vi "SMU2400Init.vi"(7 "Keithley Config":T1={"Source Compliance"=0.1, "Min Voltage"=0.0, "Max Voltage"=5.0, "Source Mode"=0, "Number of Points"=50} {"Source Mode" items=["Voltage", "Current"]}, 8 "error in (no error)":errorcluster, 11 "Keithley 2400 Name":refnum<visa-resource-name>) -> (0 "error out":errorcluster, 3 "VISA resource name out":refnum<visa-resource-name>)   [LabVIEW 2020, in "SMU.lvclass"]
uses:
  SMU.lvclass
  typeDefs/keithleySettings.ctl
  <instrlib>/Keithley 24XX/Keithley 24XX.lvlib
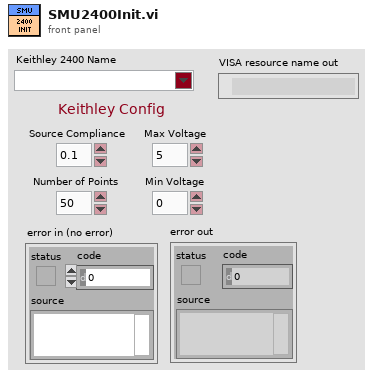
[diagram p1: front panel]
types:
  T1 = typedef "keithleySettings.ctl" = cluster{"Source Compliance":dbl, "Min Voltage":dbl, "Max Voltage":dbl, "Source Mode":u16, "Number of Points":u32}
  T2 = cluster{"Baud Rate":u32, "Parity":u16, "Data Bits":u16, "Stop Bits":u16, "Flow Control":u16}
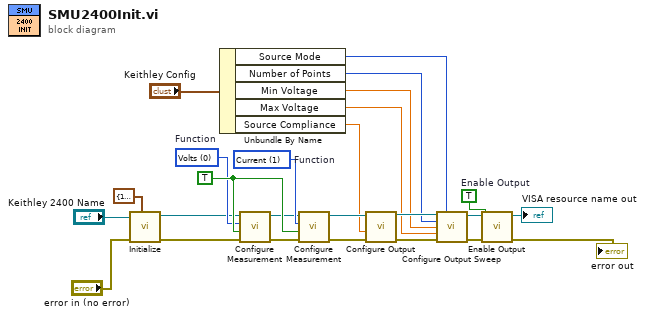
[diagram p0: block diagram]
diagram:
  w22 = TRUE  # Enable Output
  w17 = TRUE ("Enable Auto Range")
  w16 = u16 1 items=["Volts", "Current", "Resistance"]  # Function
  w15 = u16 0 items=["Volts", "Current", "Resistance"]  # Function
  n1 = call <instrlib>:"Initialize.vi"("Serial Configuration"=T2 {"Baud Rate"=19200, "Parity"=0, "Data Bits"=8, "Stop Bits"=10, "Flow Control"=0}, "error in (no error)"="error in (no error)", "VISA resource name"="Keithley 2400 Name") -> ("error out"=w12:errorcluster, "VISA resource name out"=w11:refnum<visa-resource-name>)  [unwired: 7 in]
  n2 = Unbundle By Name("Keithley Config") -> ("Source Mode"=w5:u16, "Number of Points"=w7:u32, "Min Voltage"=w8:dbl, "Max Voltage"=w9:dbl, "Source Compliance"=w4:dbl)
  n3 = call <instrlib>:"Configure Measurement.vi"("error in (no error)"=w12, "Enable Auto Range (T:Enable)"=w17, "Function (0: Volts)"=w15, "VISA resource name"=w11) -> ("error out"=w13:errorcluster, "VISA resource name out"=w14:refnum<visa-resource-name>)  [unwired: 6 in]
  n4 = call <instrlib>:"Configure Measurement.vi"("error in (no error)"=w13, "Enable Auto Range (T:Enable)"=w17, "Function (0: Volts)"=w16, "VISA resource name"=w14) -> ("error out"=w24:errorcluster, "VISA resource name out"=w23:refnum<visa-resource-name>)  [unwired: 6 in]
  n5 = call <instrlib>:"Configure Output.vi"("error in (no error)"=w24, "Compliance  Level (0.1)"=w4, "VISA resource name"=w23) -> ("error out"=w18:errorcluster, "VISA resource name out"=w19:refnum<visa-resource-name>)  [unwired: 7 in]
  n6 = call <instrlib>:"Configure Output Sweep.vi"("VISA resource name"=w19, "Source Mode  (0: Voltage)"=w5, "Number of Points (5)"=w7, "Minimum Amplitude (1)"=w8, "Maximum Amplitude (2)"=w9, "error in (no error)"=w18) -> ("VISA resource name out"=w20:refnum<visa-resource-name>, "error out"=w21:errorcluster)  [unwired: 8 in]
  n7 = call <instrlib>:"Enable Output.vi"("error in (no error)"=w21, "Enable Output (T: Enable)"=w22, "VISA resource name"=w20) -> ("error out"=→"error out":errorcluster, "VISA resource name out"=→"VISA resource name out":refnum<visa-resource-name>)  [unwired: 7 in]
